vi "tcpServerSenderLoop.vi"(8 "error in (no error)":errorcluster, 10 "notifierTcpConn":refnum<notifier>, 11 "TcpServerBase in":refnum<class "TcpServerBase.lvclass">) -> (0 "error out":errorcluster, 3 "TcpServerBase out":refnum<class "TcpServerBase.lvclass">)   [LabVIEW 2018, in "TcpServerBase.lvclass"]
doc: "Receive an ack or an event/telemetry from the LabVIEW Component to be sent to TCP Client."
uses:
  TcpServerBase.lvclass
  TcpServerBase.lvclass/TcpServerBase.ctl
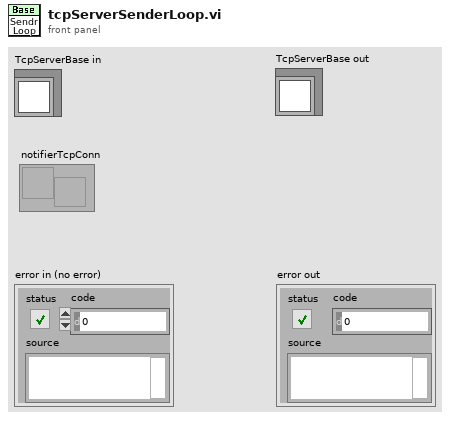
[diagram p1: front panel]
types:
  T1 = cluster{"connection ID":refnum<k5>, "firstConnection":bool}
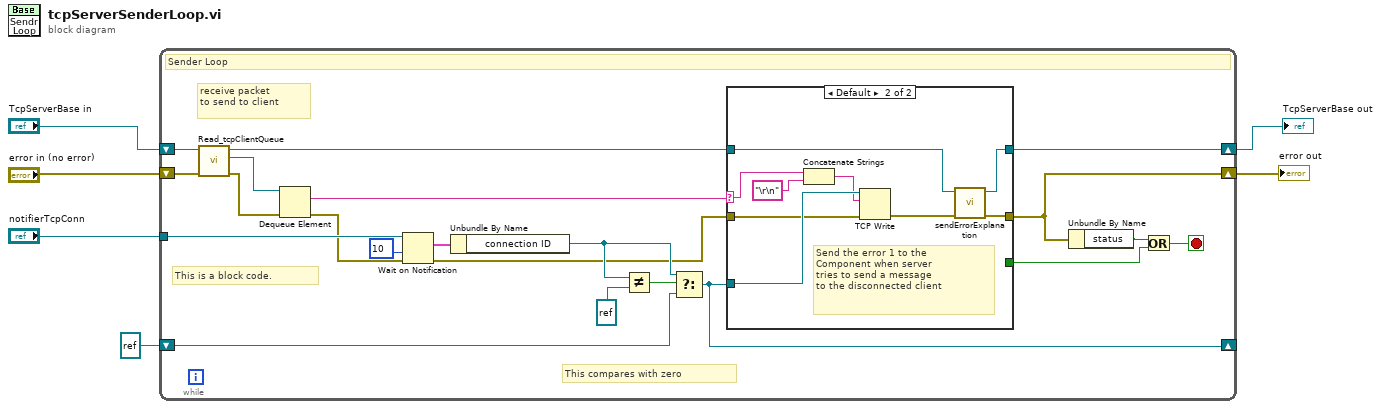
[diagram p0: block diagram]
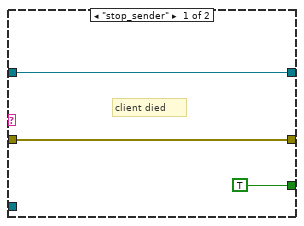
[diagram p2: hidden frame]
diagram:
  n1 = while {
    shift-right: [w21] -> w6
    shift-left: "error in (no error)" -> [w25]
    shift-right: [w18] -> w3
    shift-left: "TcpServerBase in" -> [w27]
    shift-right: [w14] -> _
    shift-left: refnum<k5> refnum ("tcpConnectionID") -> [w15]
    tunnel: "notifierTcpConn" -> [w12]
    stop <- w24 stop-if-true
    # "This compares with zero"
    # "This is a block code."
    # "receive packet\nto send to client"
    # "Sender Loop"
    n2 = call "Read_tcpClientQueue.vi"("error in (no error)"=w25, "TcpServerBase in"=w27) -> ("error out"=w19:errorcluster, "tcpClientQueue"=w26:refnum<queue>, "TcpServerBase out"=w7:refnum<class "TcpServerBase.lvclass">)  [unwired: 7 in]
    n3 = Dequeue Element(queue=w26, error in (no error)=w19) -> (element=w20:string, error out=w11:errorcluster)  [unwired: 1 in, 2 out]
    n4 = Wait on Notification(notifier=w12, timeout in ms (-1)=10, error in (no error)=w11) -> (notification=w10:T1, error out=w8:errorcluster)  [unwired: 1 in, 2 out]
    n5 = Unbundle By Name(w10) -> ("connection ID"=w9:refnum<k5>)
    n6 = Not Equal?(x=w9, y=refnum<k5> refnum ("tcpConnectionID")) -> (x != y?=w16:bool)
    n7 = Select(t=w9, s=w16, f=w15) -> (s? t:f=w14:refnum<k5>)
    n8 = case shown="Default" w20 {
      selector: w20 -> [_ w36]
      tunnel: [TRUE _] -> w23
      tunnel: [w28 w34] -> w21
      tunnel: w7 -> [w29 w33]
      tunnel: [w29 w31] -> w18
      tunnel: w14 -> [_ w39]
      tunnel: w8 -> [w28 w35]
      frame "stop_sender" {
        # "client died"
      }
      frame Default {
        # "Send the error 1 to the\nComponent when server\ntries to send a message\nto the disconnected client"
        n9 = Concatenate Strings(w36, "\r\n" ("string")) -> (w37:string)
        n10 = TCP Write(connection ID=w39, data in=w37, error in (no error)=w35) -> (error out=w32:errorcluster)  [unwired: 1 in, 2 out]
        n11 = call "sendErrorExplanation.vi"("error in (no error)"=w32, "TcpServerBase in"=w33) -> ("error out"=w34:errorcluster, "TcpServerBase out"=w31:refnum<class "TcpServerBase.lvclass">)  [unwired: 8 in]
      }
    }
    n12 = Unbundle By Name(w21) -> ("status"=w22:bool)
    n13 = Or(x=w22, y=w23) -> (x .or. y?=w24:bool)
  }
  "error out" <- w6
  "TcpServerBase out" <- w3
